vi "V7310.Main-Select.vi"(8 "error in":errorcluster, 10 "Name":string) -> (0 "error out":errorcluster, 2 "CheckDM":bool)   [LabVIEW 2016]
uses:
  tools/EventLog/EventLog.EventSource.ctl
  tools/Translator/Translator.Message.ctl
  V7310.Action.ctl
  tools/EventLog/EventLog.CreateError(array).vi
  tools/Translator/Translator.Translate.Status (NoError).vi
  tools/Translator/Translator.FormatMessage.vi
  LowLevel/V7310.Global.vi
  tools/EventLog/EventLog.CreateError(single).vi
  tools/Translator/Translator.Global.vi
  tools/ErrorHandling/ErrorHandling.Create.vi
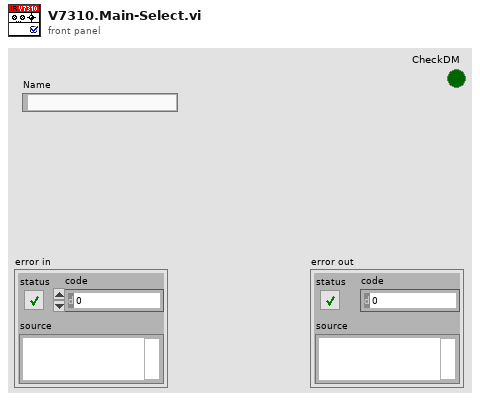
[diagram p1: front panel]
types:
  T1 = typedef "V7310.Data.Status.ctl" = cluster{"State":T2, "LaserStatus":T3, "LaserStatusRaw":string, "Ref":refnum<k5>, "RTC TS":timestamp, "Conn TS":timestamp, "Msg":T4[], "JobInUse":string, "Jobs":string[], "Vars":T5[]}
  T2 = typedef "V7310.Data.Status.State.ctl" = enum16{"First", "Init", "Msg", "Error", "Abort", "Idle", "Run"}
  T3 = typedef "V7310.LaserStatus.ctl" = enum16{"-", "FatalError", "Initialize", "KeySwitchOpen", "TimeoutInterlock", "InterlockOpen", "StartUp", "ShutterlockOpen", "Standby", "Ready", "PrepareForMarking", "WaitForTrigger", "Marking"}
  T4 = typedef "V7310.Message.Data.ctl" = cluster{"ID":i32, "Msg":string}
  T5 = typedef "V7310.Job.Variable.ctl" = cluster{"Name":string, "Value":string}
  T6 = typedef "V7310.Action.ctl" = enum32{"idle", "constructor", "destructor", "--- V7310 ---", "Init", "Select", "Start", "Stop"}
  T7 = typedef "Translator.Message.ctl" = enum16{"-", "Event confirmed", "Log out", "Log in", "Shutdown", "Cancel", "Start", "Begin time", "End time", "Duration", "Service Mode", "Ignore Results", "Serial Format", "On", "Off", "OK", "NOK", "NOK %s", "Home", "Work", "Close", "Open", "In progress...", "Missing", "Empty", "Hardware failure", "Initial", "Default", "Total", "Out of range", "Free disk space is below 1GB - contact technician", "Error %d >> %s", "Error %d >> %s >> %s", "Msg %d >> %s", "Laser msg %d %s", "Laser cmd error %s %d", "Laser cmd failed %s", "Laser cmd warning %s", "Laser disconnected", "Laser status %s", "Laser already started", "Laser job unkonwn %s", "Laser job missing %s", "Laser job select failure %s", "Unable to start laser printing (%s)", "Unable to stop laser printing (%s)", "Laser marking aborted", "Laser marking timeout", "Unable to reset Laser Interlock (%s)", "Unable to trigger Laser. Laser not ready (%s)", "Laser job '%s' coordinates not configured", "Starting %s", "Quitting %s", "Configured", "Initializing", "Quitting", "Loading", "Loaded %d results", "Loaded %d events", "Running", "Stopped", "Summary", "Laser", "Do you want to continue?", "Do you want to delete the configuration?", "The configuration is being used by an order. Unable to delete!", "Press confirm button", "Station is not based. Do you want to exit?", "Station requires changeover. Do you want to run the test?", "Test options are not set as default. Do you want to continue?", "Product not detected. Do you want to continue?", "Product scan failed. Do you want to continue?", "Calibration", "Log out?", "System", "All", "IDLE", "Translating...%s", "Not found", "Alarm %s", "Run", "Skip", "Abort", "Repeat", "Please wait...", "Database disconnected", "Database disconnected - changeover disabled!", "Login to database successful", "Login to database failed: %d; %s", "Unable to check the product status of reference %d - database disconnected", "Unable to set the product status of reference %d - database disconnected", "Variant file backup %s", "Read variant (%s)", "Result", "Station armed!", "Station requires changeover!", "Select reference number...", "EMERGENCY BUTTON - press Control button", "EMERGENCY DOOR - press Control button", "Resetting Emergency...", "Unable to reset safety circuit - Emergency Button pressed", "Unable to reset safety circuit - Emergency Side Door open", "Station not based", "Station based", "Station not empty", "Station basing...", "No order", "Press Start to begin new order", "Scanning new order", "Order NOK. Correct or scan again", "Order OK. Press Accept", "Order ready", "Revolver incorrect", "Fork incorrect", "Revolver missing", "Revolver empty", "Container missing", "Offline results", "Offline statistics", "Updating statistics %.1f %%", "DMC Configurator", "Door open", "Close the front door", "Press start button", "Done. Open the front door", "Running...", "Running...%.1f %%", "Pause %s", "Pause %s. NOK container missing", "Pause %s. OK container missing", "Pause %s. Revolver empty", "Pause %s. Revolver missing", "Pause %s. Revolver incorrect", "Pause %s. Fork missing", "Pause %s. Fork incorrect", "Pause %s. Too many failures", "Pause %s. One slot is not working", "Pause %s. Part order is done. Empty OK container", "Pause %s. Unable to move product to slot", "Pause %s. Unable to move back product pusher", "Pause %s. Unable to lift product", "Pause %s. Unable to move back product lifter", "Pause %s. Unable to move product arm to Work", "Pause %s. Unable to move product arm to NOK", "Pause %s. Unable to move product arm to OK", "Pause %s. Unable to unsuck the NOK product", "Pause %s. Unable to drop the NOK product", "Pause %s. Product OK missing", "Pause %s. Unable to unsuck the OK product", "Pause %s. Unable to drop the OK product", "Stopping...", "File '%s' is missing", "File '%s' is broken", "File '%s' is running", "Log file started (%s)", "Log file ended (%s)", "Log file stopped (%s)", "Log file ignored (%s)", "Log file exported (%s)", "Log file export failed (%s)", "Wrong serial number in log file", "Wrong reference number in log file", "Test steps are missing", "%s = %.3f", "Process param '%s' not found in DB", "Process param '%s' wrong order", "Process param '%s' value %.3f out of limits (%.3f; %.3f)", "Step%d param '%s' not found in DB", "Step%d param '%s' wrong order", "Step%d param '%s' value %.3f out of limits (%.3f; %.3f)", "Step%d EV '%s' not found in DB", "Step%d EV '%s' wrong order", "\"%s\" not found in DB", "\"%s\" wrong order", "\"%s\" value %.3f out of limits (%.3f; %.3f)", "\"%s\" not found in software", "Process init (%s)", "Process started", "Process restarted", "Process run", "Process done", "Process aborted", "Process aborted at work", "Process aborted at home", "Process error", "Process error at home", "Process error at work", "Process close", "Select plate from the order to process", "Do you want to start the process?", "Do you want to continue the process?", "There is unfinished order. Do you want to put the new order?", "Product %s %d OK", "Product %s %d NOK", "Unable to unload the slot %s. Product missing in the slot", "Unable to unload the slot %s. Product already in the arm", "Unable to accept the product as OK. Product missing in slot %s", "Unable to accept the product as OK. Product could not drop into the container at slot %s", "Unable to accept the product as NOK. Product could not drop into the container at slot %s", "Scan failed. Error %s", "Scan failed. Scanner disconnected", "Scan failed. Wrong Wabco number %d, limit (%d,%d)", "Scan failed. Wrong serial number %d, limit (%d,%d)", "Scan failed. Wrong date %d, limit (%d,%d)", "Scan failed. Wrong product wabco number %d (expected %d)", "Scan failed. Wrong product serial number %d (expected > 0)", "Scan OK %s", "Scan failed. Unable to determine table position (%s)", "Scan failed. Timeout", "Tune failed. Scanner disconnected", "Tune failed. Timeout", "%s = %d", "%s = %d->%d", "Unable to set %s = %.2f - Air Pressure Inside off", "Unable to set digital output '%s' = %d", "Unable to activate air pressure inside - timeout", "Unable to activate air pressure inside - aborted", "Unable to switch on Air Main Valve - Air Pressure Inlet off", "Unable to switch on Air Main Valve - Door open", "Unable to switch off Air Main Valve - timeout", "Unable to switch off Air Main Valve - aborted", "Unable to rotate Table - timeout", "Unable to rotate Table - aborted", "Unable to rotate Table - Product Move not in Home position", "Unable to rotate Table - Air Pressure Inside off", "Unable to rotate Table - Product Lift A not in Home position", "Unable to rotate Table - Product Lift B not in Home position", "Unable to rotate Table - unlock before movement timeout", "Unable to rotate Table - lock after movement timeout", "Unable to move Table Lock to %s position - timeout", "Unable to move Table Lock to %s position - aborted", "Unable to move Table Lock to %s position - Air Pressure Inside off", "Unable to move Table Lock to %s position - Table not in position", "Unable to move Product Lift A to %s position - timeout", "Unable to move Product Lift B to %s position - timeout", "Unable to move Product Lift A to %s position - aborted", "Unable to move Product Lift B to %s position - aborted", "Unable to move Product Lift A to %s position - Air Pressure Inside off", "Unable to move Product Lift B to %s position - Air Pressure Inside off", "Unable to move Product Lift A to %s position - Table not locked", "Unable to move Product Lift B to %s position - Table not locked", "Unable to move Product Lift A to %s position - Product Arm not in Work position", "Unable to move Product Lift B to %s position - Product Arm not in Work position", "Unable to set Product Suction Gripper %s to %s - timeout", "Unable to set Product Suction Gripper %s to %s - aborted", "Unable to set Product Suction Gripper %s to %s - Air Pressure Inside off", "Unable to set Product Suction Gripper %s to %s - Table slot unkown", "Unable to move Product Arm to %s position - timeout", "Unable to move Product Arm to %s position - aborted", "Unable to move Product Arm to %s position - Air Pressure Inside off", "Unable to move Product Arm to %s position - Product Lift A not in Home position", "Unable to move Product Arm to %s position - Product Lift B not in Home position", "Unable to move Product to %s position - timeout", "Unable to move Product to %s position - aborted", "Unable to move Product to %s position - Air Pressure Inside off", "Unable to move Product to %s position - Table not in position"}
  T8 = typedef "EventLog.EventSource.ctl" = enum16{"All", "Gui", "Ref", "File", "Arch", "Seq", "CPX", "DB", "Laser", "Scan.P", "Scan.O"}
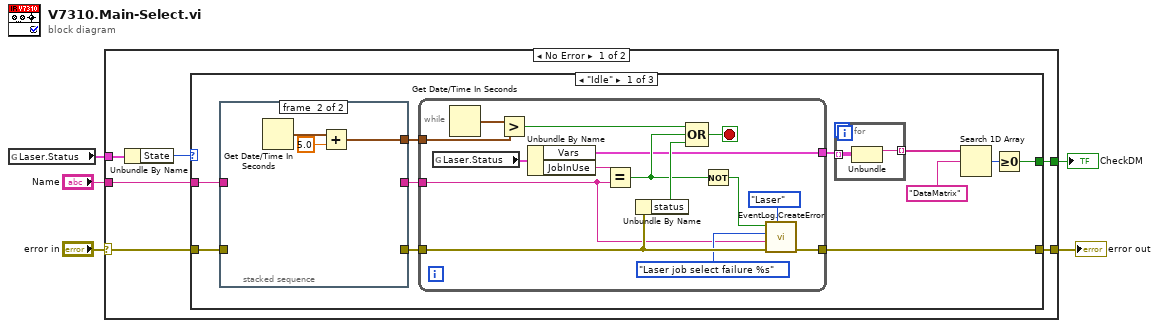
[diagram p0: block diagram]
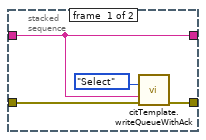
[diagram p2: hidden frame]
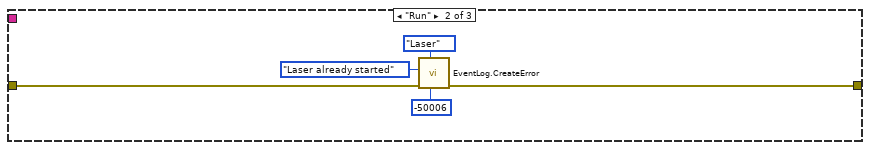
[diagram p3: hidden frame]
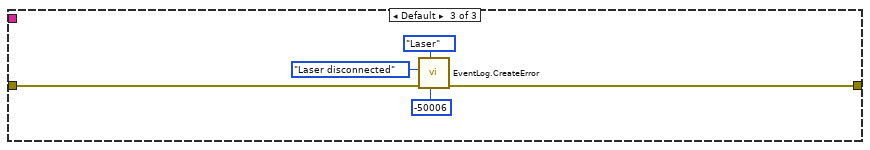
[diagram p4: hidden frame]
diagram:
  n1 = global read "V7310.Global.vi" "Laser.Status"() -> (w2:T1)
  n2 = case shown="No Error" "error in" {
    selector: "error in" -> [w11 w57]
    tunnel: [w9 w57] -> w4
    tunnel: "Name" -> [w10 _]
    tunnel: w2 -> [w8 _]
    tunnel: [w6 _] -> w1
    frame No Error {
      n3 = Unbundle By Name(w8) -> ("State"=w7:T2)
      n4 = case shown="\"Idle\"" w7 {
        tunnel: w11 -> [w22 w48 w53]
        tunnel: w10 -> [w21 _ _]
        tunnel: [w19 w47 w52] -> w9
        tunnel: [w13 _ _] -> w6
        frame "Idle" {
          n5 = stacked-sequence {
            tunnel: w22 -> [w25 _]
            tunnel: w21 -> [w26 _]
            tunnel: [w27 _] -> w20
            tunnel: [w26 _] -> w18
            tunnel: [_ w29] -> w17
            frame #0 {
              n6 = call "citTemplate.writeQueueWithAck.vi"("event in"=V7310.Action."Select" ("Action"), "(flatten) data in"=w26, "error in (no error)"=w25) -> ("error out"=w27:errorcluster)  [unwired: 10 in, 2 out]
            }
            frame #1 {
              n7 = Get Date/Time In Seconds() -> (seconds since 1Jan1904=w31:timestamp)
              n8 = Add(x=w31, y=5.0) -> (x+y=w29:timestamp)
            }
          }
          n9 = while {
            tunnel: w20 -> [w38]
            tunnel: [w37] -> w19
            tunnel: w18 -> [w33]
            tunnel: w17 -> [w44]
            tunnel: [w32] -> w14
            stop <- w40 stop-if-true
            n10 = global read "V7310.Global.vi" "Laser.Status"() -> (w46:T1)
            n11 = Get Date/Time In Seconds() -> (seconds since 1Jan1904=w45:timestamp)
            n12 = Greater?(x=w45, y=w44) -> (0:w42:bool)
            n13 = Unbundle By Name(w46) -> ("Vars"=w32:T5[], "JobInUse"=w43:string)
            n14 = Equal?(x=w43, y=w33) -> (x = y?=w35:bool)
            n15 = Unbundle By Name(w38) -> ("status"=w41:bool)
            n16 = Compound Arithmetic op=OR(w42, w35, w41) -> (w40:bool)
            n17 = Not(x=w35) -> (.not. x?=w34:bool)
            n18 = call-poly "EventLog.CreateError.vi"("Source (All)"=EventLog.EventSource."Laser", "error in"=w38, "arg"=w33, "msg"=Translator.Message."Laser job select failure %s", "create (T)"=w34) -> ("error out"=w37:errorcluster)  [unwired: 6 in]
          }
          n19 = for {
            tunnel: w14 -> [w24] mode=indexing
            tunnel: [w23] -> w16 mode=indexing
            n20 = Unbundle(w24) -> ("Name"=w23:string)  [unwired: 1 out]
          }
          n21 = Search 1D Array(1D array=w16, element="DataMatrix") -> (index of element=w15:i32)  [unwired: 1 in]
          n22 = Greater Or Equal To 0?(x=w15) -> (x >= 0?=w13:bool)
        }
        frame "Run" {
          n23 = call-poly "EventLog.CreateError.vi"("Code (-1)"=-50006 ("error code (0)"), "Source (All)"=EventLog.EventSource."Laser", "error in"=w48, "msg"=Translator.Message."Laser already started") -> ("error out"=w47:errorcluster)  [unwired: 6 in, 1 out]
        }
        frame Default {
          n24 = call-poly "EventLog.CreateError.vi"("Code (-1)"=-50006 ("error code (0)"), "Source (All)"=EventLog.EventSource."Laser", "error in"=w53, "msg"=Translator.Message."Laser disconnected") -> ("error out"=w52:errorcluster)  [unwired: 6 in, 1 out]
        }
      }
    }
    frame Error {
    }
  }
  "error out" <- w4
  "CheckDM" <- w1
